vi "Read DMA and Update Waveform.vi"(4 "Delacing Scheme":T3, 6 "Number of Channels":u8, 7 "Timeout?":bool, 8 "error in (no error)":errorcluster, 9 "Total Samples":u32, 10 "Refs in":T1={"Data Type"=enum."Boolean", "DMA_SGL"=refnum, "DMA_U64"=refnum, "DMA_I64"=refnum, "DMA_FXP+/-32.8"=refnum, "DMA_FXP+/-64.32"=refnum, "DMA_U32"=refnum, "DMA_U16"=refnum, "DMA_U8"=refnum, "DMA_I32"=refnum, "DMA_I16"=refnum, "DMA_I8"=refnum, "DMA_FXP+/-32.16"=refnum} {"Data Type" format="%.0x"}, 11 "Multiple Waveforms Write (DBL) in":refnum<class "Multiple Waveforms Write (DBL).lvclass">) -> (0 "error out":errorcluster, 1 "Elements Remaining":u32, 2 "Refs in":T1={"Data Type"=enum."Boolean", "DMA_SGL"=refnum, "DMA_U64"=refnum, "DMA_I64"=refnum, "DMA_FXP+/-32.8"=refnum, "DMA_FXP+/-64.32"=refnum, "DMA_U32"=refnum, "DMA_U16"=refnum, "DMA_U8"=refnum, "DMA_I32"=refnum, "DMA_I16"=refnum, "DMA_I8"=refnum, "DMA_FXP+/-32.16"=refnum} {"Data Type" format="%.0x"}, 3 "Multiple Waveforms Write (DBL) out":refnum<class "Multiple Waveforms Write (DBL).lvclass">)   [LabVIEW 2020, in "FPGA Addon Engine.lvlib"]
uses:
  FPGA Addon Engine.lvlib
  Addon Shared/Types/Delacing Scheme.ctl
  Types/DMA Input Refs.ctl
  Addon Shared/Types/FPGA Addon Data Type.ctl
  <vilib>/NI VeriStand/Custom Device Waveform API/Multiple Waveforms Write (DBL)/Multiple Waveforms Write (DBL).lvclass
  C:/Program Files (x86)/National Instruments/LabVIEW 2020/vi.lib/NI VeriStand/Custom Device Waveform API/Waveform Session.lvclass
  <vilib>/NI VeriStand/Custom Device Waveform API/Waveform Session.lvclass/Waveform Session.ctl
  <vilib>/NI VeriStand/Custom Device Waveform API/Multiple Waveforms Write (DBL)/Multiple Waveforms Write (DBL).lvclass/Multiple Waveforms Write (DBL).ctl
  <vilib>/NI VeriStand/Custom Device Waveform API/Internal Comm Classes/WPL Comm/WPL Comm (2D DBL)/WPL Comm (2D DBL).lvclass/WPL Comm (2D DBL).ctl
  <vilib>/NI VeriStand/Custom Device Waveform API/Internal Comm Classes/WPL Comm/WPL Comm.lvclass/WPL Comm.ctl
  <vilib>/NI VeriStand/Custom Device Waveform API/Multiple Waveforms Write (DBL)/NI VeriStand - Write Multiple Waveforms (DBL).vi
  <vilib>/NI VeriStand/Custom Device Waveform API/Read Sample offset DVR.vi
  <vilib>/NI VeriStand/Custom Device Waveform API/Internal Comm Classes/WPL Comm/WPL Comm (2D DBL)/Comm_write 2d dbl.vi
  <vilib>/NI VeriStand/Custom Device Waveform API/Check Write Size.vi
  <vilib>/NI VeriStand/Custom Device Waveform API/Check Opened.vi
  <vilib>/NI VeriStand/Custom Device Waveform API/Internal Comm Classes/WPL Comm/Direct Send WPL Command.vi
  <vilib>/NI VeriStand/Custom Device Waveform API/Internal Comm Classes/WPL Comm/Convert Q Error to Shutdown Error.vi
  <vilib>/NI VeriStand/Custom Device Waveform API/Internal Comm Classes/WPL Comm/WPL Comm (2D DBL)/WPL Comm (2D DBL).lvclass
  C:/Program Files (x86)/National Instruments/LabVIEW 2020/vi.lib/NI VeriStand/Custom Device Waveform API/Internal Comm Classes/WPL Comm/WPL Comm.lvclass
  <vilib>/Utility/error.llb/Error Cluster From Error Code.vi
  <vilib>/rvi/errors/niLvFpgaAdjustHostInterfaceError.vi
  <vilib>/rvi/interface/nirviMethod/nirviMethod.xnode
  <vilib>/NI VeriStand/Custom Device Waveform API/NI_VS Custom Device Waveform API.lvlib
  <vilib>/FPGAPlugInAG/Dynamic/niLvFpga_ReadFifo_Dynamic.vi
  <vilib>/rvi/errors/niLvFpgaMergeErrorWithErrorCode.vi
  Addon Shared/FPGA Addon Shared.lvlib
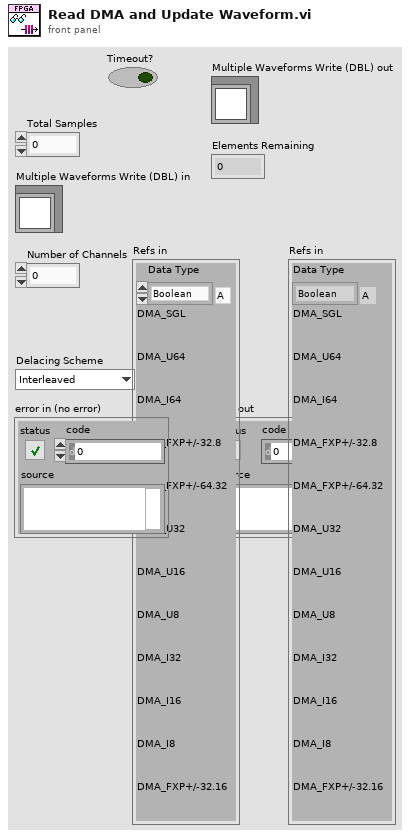
[diagram p1: front panel]
types:
  T1 = typedef "FPGA Addon Engine.lvlib/DMA Input Refs.ctl" = cluster{"Data Type":T2, "DMA_SGL":refnum<k20>, "DMA_U64":refnum<k20>, "DMA_I64":refnum<k20>, "DMA_FXP+/-32.8":refnum<k20>, "DMA_FXP+/-64.32":refnum<k20>, "DMA_U32":refnum<k20>, "DMA_U16":refnum<k20>, "DMA_U8":refnum<k20>, "DMA_I32":refnum<k20>, "DMA_I16":refnum<k20>, "DMA_I8":refnum<k20>, "DMA_FXP+/-32.16":refnum<k20>}
  T2 = typedef "FPGA Addon Shared.lvlib/FPGA Addon Data Type.ctl" = enum8{"<Null>", "I8", "I16", "I32", "I64", "U8", "U16", "U32", "U64", "SGL", "Boolean", "Analog PWM In Settings", "Analog PWM In", "Digital PWM In Settings", "Digital PWM In", "Digital PWM Out", "Sine Out", "FXP", "FXP+/-24.5", "FXP+/-16.5", "FXP+/-32.8", "FXP+/-64.32", "FXP+/-16.7", "FXP+/-20.5", "FXP+/-27.5", "FXP+/-32.16", "FXP+16.3", "FXP+18.3", "Digital Static In", "Digital Static Out", "Digital Static In Settings", "Digital WSS Out", "Quad Encoder Settings", "Quad Encoder In", "Group"}
  T3 = typedef "FPGA Addon Shared.lvlib/Delacing Scheme.ctl" = enum8{"Interleaved", "Bitpacked"}
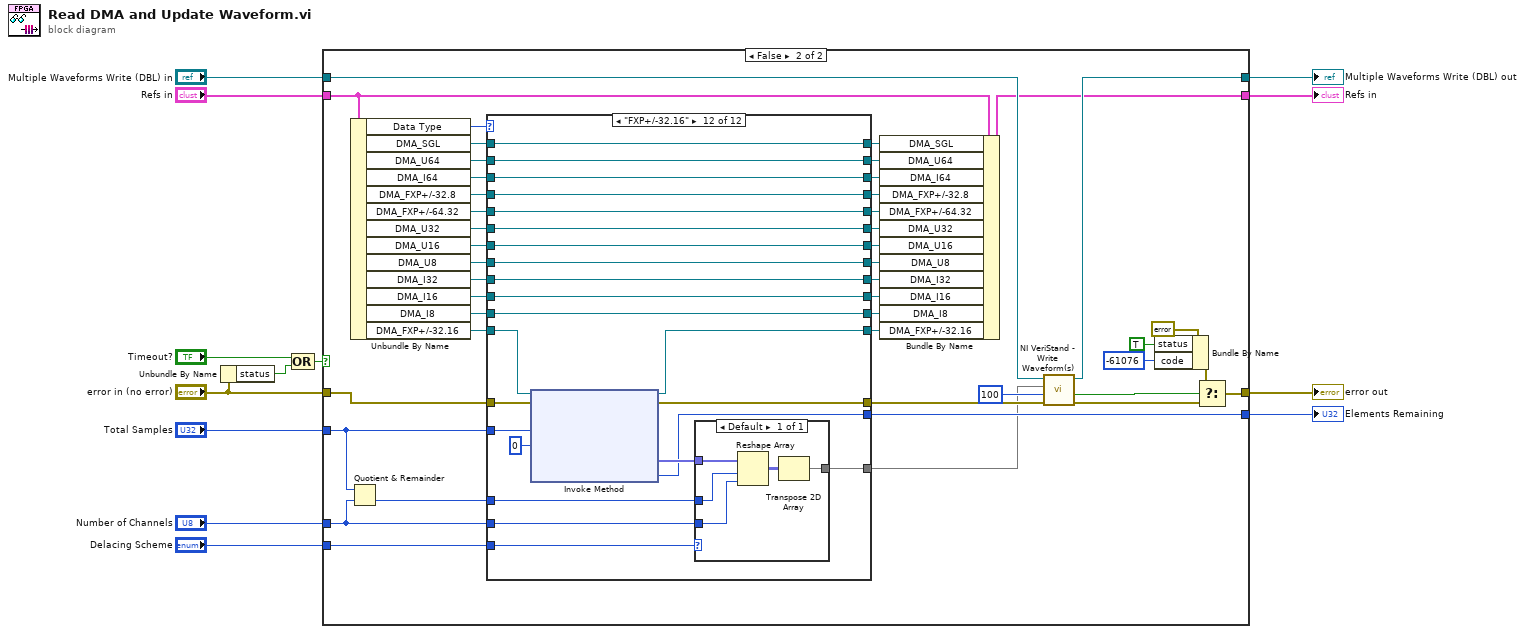
[diagram p0: block diagram]
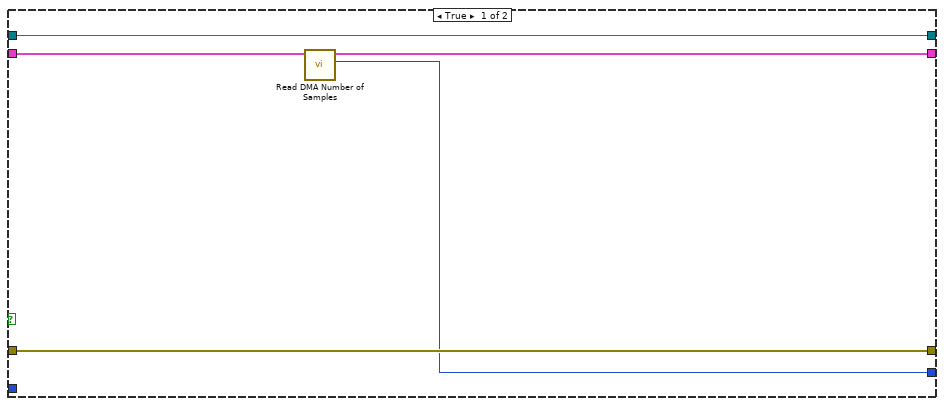
[diagram p2: hidden frame]
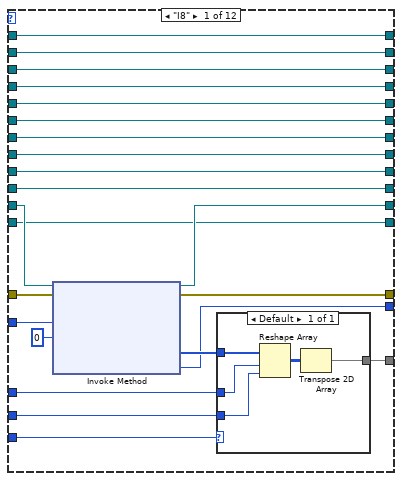
[diagram p3: hidden frame]
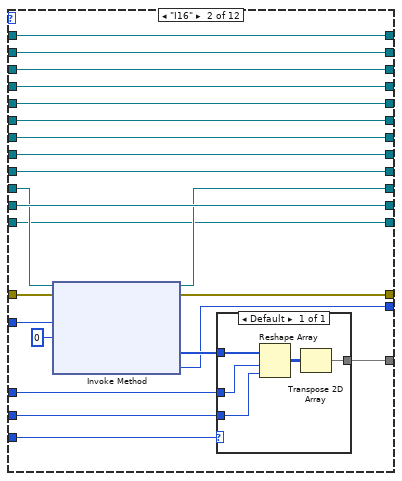
[diagram p4: hidden frame]
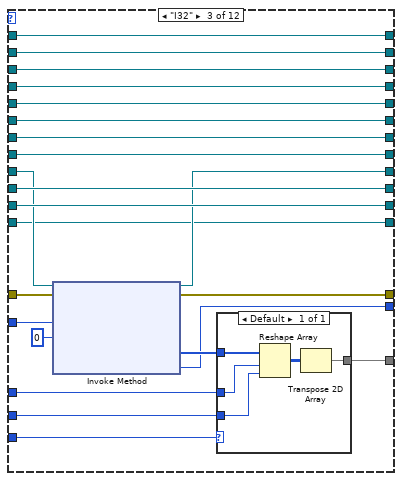
[diagram p5: hidden frame]
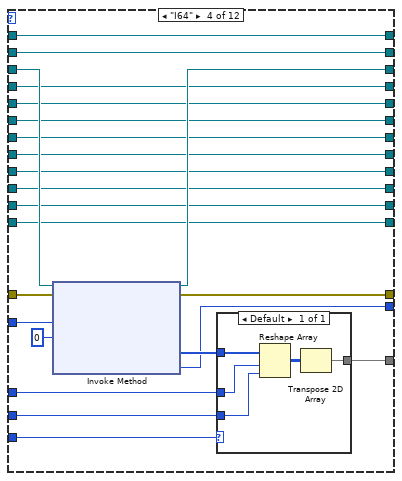
[diagram p6: hidden frame]
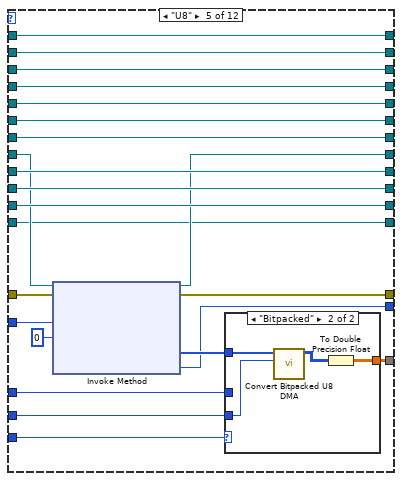
[diagram p7: hidden frame]
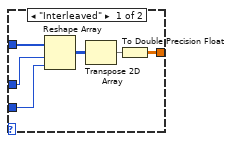
[diagram p8: hidden frame]
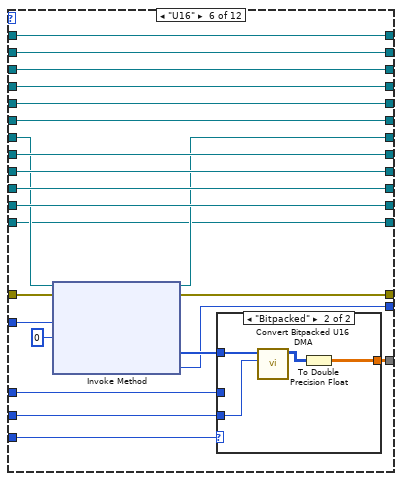
[diagram p9: hidden frame]
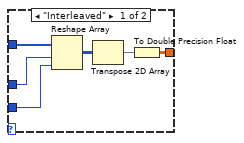
[diagram p10: hidden frame]
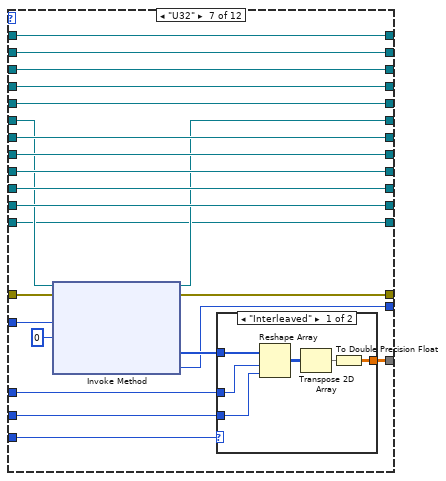
[diagram p11: hidden frame]
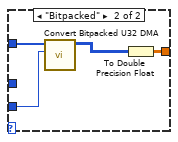
[diagram p12: hidden frame]
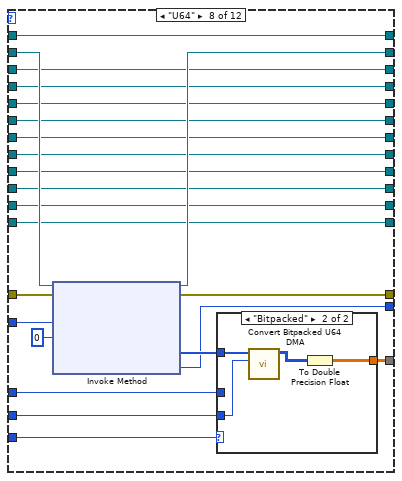
[diagram p13: hidden frame]
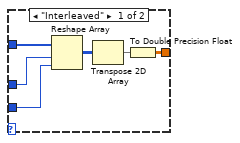
[diagram p14: hidden frame]
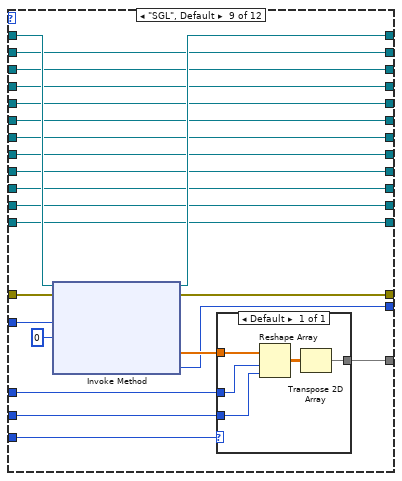
[diagram p15: hidden frame]
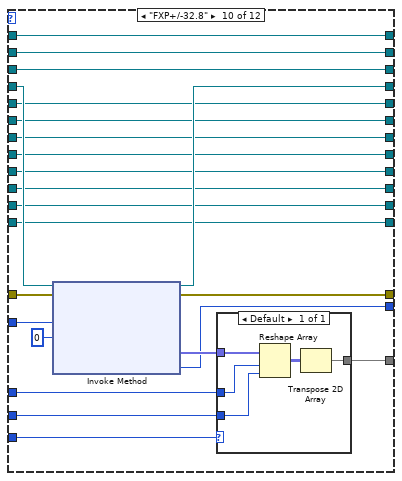
[diagram p16: hidden frame]
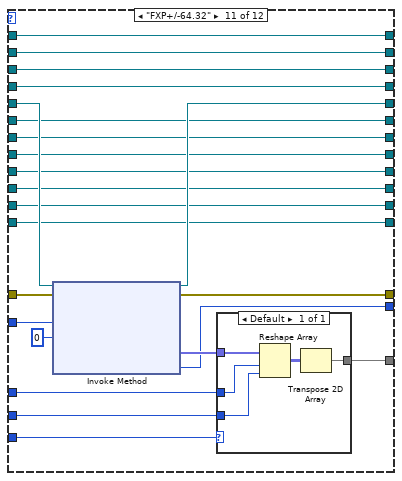
[diagram p17: hidden frame]
diagram:
  n1 = Unbundle By Name("error in (no error)") -> ("status"=w3:bool)
  n2 = Compound Arithmetic op=OR("Timeout?", w3) -> (w1:bool)
  n3 = case shown="False" w1 {
    tunnel: [w17 w63] -> w13
    tunnel: [w16 w56] -> w12
    tunnel: "Delacing Scheme" -> [_ w54]
    tunnel: [w14 w41] -> w10
    tunnel: "Refs in" -> [w15 w42]
    tunnel: [w18 w53] -> w8
    tunnel: "Multiple Waveforms Write (DBL) in" -> [w18 w50]
    tunnel: "Total Samples" -> [_ w49]
    tunnel: "Number of Channels" -> [_ w48]
    tunnel: "error in (no error)" -> [w17 w46]
    frame True {
      n4 = call "Read DMA Number of Samples.vi"("Refs in"=w15) -> ("Elements Remaining"=w16:u32, "Refs out"=w14:T1)  [unwired: 8 in, 1 out]
    }
    frame False {
      n5 = Quotient & Remainder(x=w49, y=w48) -> (floor(x/y)=w47:u32)  [unwired: 1 out]
      n6 = Unbundle By Name(w42) -> ("Data Type"=w45:T2, "DMA_SGL"=w44:refnum<k20>, "DMA_U64"=w43:refnum<k20>, "DMA_I64"=w38:refnum<k20>, "DMA_FXP+/-32.8"=w36:refnum<k20>, "DMA_FXP+/-64.32"=w33:refnum<k20>, "DMA_U32"=w21:refnum<k20>, "DMA_U16"=w24:refnum<k20>, "DMA_U8"=w25:refnum<k20>, "DMA_I32"=w28:refnum<k20>, "DMA_I16"=w29:refnum<k20>, "DMA_I8"=w32:refnum<k20>, "DMA_FXP+/-32.16"=w20:refnum<k20>)
      n7 = case shown="\"FXP+/-32.16\"" w45 {
        tunnel: [w85 w113 w141 w169 w197 w230 w263 w296 w329 w357 w385 w413] -> w56
        tunnel: w54 -> [w84 w112 w140 w168 w196 w229 w262 w295 w328 w356 w384 w412]
        tunnel: [w76 w104 w132 w160 w189 w221 w254 w287 w327 w348 w376 w404] -> w40
        tunnel: [w83 w111 w139 w167 w177 w228 w261 w294 w326 w355 w383 w411] -> w52
        tunnel: [w82 w110 w138 w166 w195 w227 w260 w293 w325 w354 w382 w410] -> w51
        tunnel: w49 -> [w80 w108 w136 w164 w193 w225 w258 w291 w323 w352 w380 w408]
        tunnel: w48 -> [w79 w107 w135 w163 w192 w224 w257 w290 w322 w351 w379 w407]
        tunnel: w47 -> [w78 w106 w134 w162 w191 w223 w256 w289 w321 w350 w378 w406]
        tunnel: w46 -> [w77 w105 w133 w161 w190 w222 w255 w288 w320 w349 w377 w405]
        tunnel: w44 -> [w76 w104 w132 w160 w189 w221 w254 w287 w319 w348 w376 w404]
        tunnel: w43 -> [w67 w95 w123 w157 w180 w212 w245 w286 w318 w347 w375 w403]
        tunnel: [w67 w95 w123 w157 w180 w212 w245 w285 w318 w347 w375 w403] -> w39
        tunnel: w38 -> [w75 w103 w131 w159 w188 w220 w253 w284 w317 w346 w372 w401]
        tunnel: [w75 w103 w131 w158 w188 w220 w253 w284 w317 w346 w372 w401] -> w37
        tunnel: w36 -> [w74 w102 w130 w156 w187 w219 w252 w283 w316 w345 w374 w402]
        tunnel: [w74 w102 w130 w156 w187 w219 w252 w283 w316 w344 w374 w402] -> w35
        tunnel: [w73 w101 w129 w155 w186 w218 w251 w282 w315 w343 w371 w392] -> w34
        tunnel: w33 -> [w73 w101 w129 w155 w186 w218 w251 w282 w315 w343 w373 w392]
        tunnel: w32 -> [w66 w96 w124 w149 w181 w213 w246 w276 w314 w337 w365 w395]
        tunnel: [w65 w96 w124 w149 w181 w213 w246 w276 w314 w337 w365 w395] -> w31
        tunnel: [w68 w93 w125 w150 w182 w214 w247 w277 w313 w338 w366 w396] -> w30
        tunnel: w29 -> [w68 w94 w125 w150 w182 w214 w247 w277 w313 w338 w366 w396]
        tunnel: w28 -> [w69 w97 w122 w151 w183 w215 w248 w278 w312 w339 w367 w397]
        tunnel: [w69 w97 w121 w151 w183 w215 w248 w278 w312 w339 w367 w397] -> w27
        tunnel: [w70 w98 w126 w152 w178 w216 w249 w279 w311 w340 w368 w398] -> w26
        tunnel: w25 -> [w70 w98 w126 w152 w179 w216 w249 w279 w311 w340 w368 w398]
        tunnel: w24 -> [w71 w99 w127 w153 w184 w211 w250 w280 w310 w341 w369 w399]
        tunnel: [w71 w99 w127 w153 w184 w210 w250 w280 w310 w341 w369 w399] -> w23
        tunnel: [w72 w100 w128 w154 w185 w217 w243 w281 w309 w342 w370 w400] -> w22
        tunnel: w21 -> [w72 w100 w128 w154 w185 w217 w244 w281 w309 w342 w370 w400]
        tunnel: w20 -> [w64 w92 w120 w148 w176 w209 w242 w275 w308 w336 w364 w394]
        tunnel: [w64 w92 w120 w148 w176 w209 w242 w275 w308 w336 w364 w393] -> w19
        frame "I8" {
          n8 = xnode "Invoke Method"("FPGA VI Reference In"=w66, "error in"=w77, "Number of Elements"=w80, "Timeout (ms)"=0) -> ("FPGA VI Reference Out"=w65:refnum<k20>, "error out"=w83:errorcluster, "Data"=w86:i8[], "Elements Remaining"=w85:u32)
          n9 = case shown="Default" w84 {
            tunnel: w86 -> [w90]
            tunnel: [w89] -> w82
            tunnel: w79 -> [w88]
            tunnel: w78 -> [w87]
            frame Default {
              n10 = Reshape Array(w90, w87, w88) -> (w91:i8[][])
              n11 = Transpose 2D Array(2D array=w91) -> (transposed array=w89:i8[][])
            }
          }
        }
        frame "I16" {
          n12 = xnode "Invoke Method"("FPGA VI Reference In"=w94, "error in"=w105, "Number of Elements"=w108, "Timeout (ms)"=0) -> ("FPGA VI Reference Out"=w93:refnum<k20>, "error out"=w111:errorcluster, "Data"=w114:i16[], "Elements Remaining"=w113:u32)
          n13 = case shown="Default" w112 {
            tunnel: w114 -> [w118]
            tunnel: [w117] -> w110
            tunnel: w107 -> [w116]
            tunnel: w106 -> [w115]
            frame Default {
              n14 = Reshape Array(w118, w115, w116) -> (w119:i16[][])
              n15 = Transpose 2D Array(2D array=w119) -> (transposed array=w117:i16[][])
            }
          }
        }
        frame "I32" {
          n16 = xnode "Invoke Method"("FPGA VI Reference In"=w122, "error in"=w133, "Number of Elements"=w136, "Timeout (ms)"=0) -> ("FPGA VI Reference Out"=w121:refnum<k20>, "error out"=w139:errorcluster, "Data"=w142:i32[], "Elements Remaining"=w141:u32)
          n17 = case shown="Default" w140 {
            tunnel: w142 -> [w146]
            tunnel: [w145] -> w138
            tunnel: w135 -> [w144]
            tunnel: w134 -> [w143]
            frame Default {
              n18 = Reshape Array(w146, w143, w144) -> (w147:i32[][])
              n19 = Transpose 2D Array(2D array=w147) -> (transposed array=w145:i32[][])
            }
          }
        }
        frame "I64" {
          n20 = xnode "Invoke Method"("FPGA VI Reference In"=w159, "error in"=w161, "Number of Elements"=w164, "Timeout (ms)"=0) -> ("FPGA VI Reference Out"=w158:refnum<k20>, "error out"=w167:errorcluster, "Data"=w170:i64[], "Elements Remaining"=w169:u32)
          n21 = case shown="Default" w168 {
            tunnel: w170 -> [w174]
            tunnel: [w173] -> w166
            tunnel: w163 -> [w172]
            tunnel: w162 -> [w171]
            frame Default {
              n22 = Reshape Array(w174, w171, w172) -> (w175:i64[][])
              n23 = Transpose 2D Array(2D array=w175) -> (transposed array=w173:i64[][])
            }
          }
        }
        frame "U8" {
          n24 = xnode "Invoke Method"("FPGA VI Reference In"=w179, "error in"=w190, "Number of Elements"=w193, "Timeout (ms)"=0) -> ("FPGA VI Reference Out"=w178:refnum<k20>, "error out"=w177:errorcluster, "Data"=w198:u8[], "Elements Remaining"=w197:u32)
          n25 = case shown="\"Bitpacked\"" w196 {
            tunnel: w198 -> [w203 w208]
            tunnel: [w199 w205] -> w195
            tunnel: w192 -> [w201 w206]
            tunnel: w191 -> [w200 _]
            frame "Interleaved" {
              n26 = Reshape Array(w203, w200, w201) -> (w204:u8[][])
              n27 = Transpose 2D Array(2D array=w204) -> (transposed array=w202:u8[][])
              n28 = To Double Precision Float(number=w202) -> (double precision float=w199:dbl[][])
            }
            frame "Bitpacked" {
              n29 = call "Convert Bitpacked U8 DMA.vi"("Channels"=w206, "binary array"=w208) -> ("Data"=w207:u8[][])  [unwired: 9 in]
              n30 = To Double Precision Float(number=w207) -> (double precision float=w205:dbl[][])
            }
          }
        }
        frame "U16" {
          n31 = xnode "Invoke Method"("FPGA VI Reference In"=w211, "error in"=w222, "Number of Elements"=w225, "Timeout (ms)"=0) -> ("FPGA VI Reference Out"=w210:refnum<k20>, "error out"=w228:errorcluster, "Data"=w231:u16[], "Elements Remaining"=w230:u32)
          n32 = case shown="\"Bitpacked\"" w229 {
            tunnel: w231 -> [w236 w241]
            tunnel: [w232 w239] -> w227
            tunnel: w224 -> [w234 w238]
            tunnel: w223 -> [w233 _]
            frame "Interleaved" {
              n33 = Reshape Array(w236, w233, w234) -> (w237:u16[][])
              n34 = Transpose 2D Array(2D array=w237) -> (transposed array=w235:u16[][])
              n35 = To Double Precision Float(number=w235) -> (double precision float=w232:dbl[][])
            }
            frame "Bitpacked" {
              n36 = call "Convert Bitpacked U16 DMA.vi"("Channels"=w238, "binary array"=w241) -> ("Data"=w240:u8[][])  [unwired: 9 in]
              n37 = To Double Precision Float(number=w240) -> (double precision float=w239:dbl[][])
            }
          }
        }
        frame "U32" {
          n38 = xnode "Invoke Method"("FPGA VI Reference In"=w244, "error in"=w255, "Number of Elements"=w258, "Timeout (ms)"=0) -> ("FPGA VI Reference Out"=w243:refnum<k20>, "error out"=w261:errorcluster, "Data"=w264:u32[], "Elements Remaining"=w263:u32)
          n39 = case shown="\"Interleaved\"" w262 {
            tunnel: w264 -> [w269 w273]
            tunnel: [w265 w274] -> w260
            tunnel: w257 -> [w267 w272]
            tunnel: w256 -> [w266 _]
            frame "Interleaved" {
              n40 = Reshape Array(w269, w266, w267) -> (w270:u32[][])
              n41 = Transpose 2D Array(2D array=w270) -> (transposed array=w268:u32[][])
              n42 = To Double Precision Float(number=w268) -> (double precision float=w265:dbl[][])
            }
            frame "Bitpacked" {
              n43 = call "Convert Bitpacked U32 DMA.vi"("Channels"=w272, "binary array"=w273) -> ("Data"=w271:u8[][])  [unwired: 9 in]
              n44 = To Double Precision Float(number=w271) -> (double precision float=w274:dbl[][])
            }
          }
        }
        frame "U64" {
          n45 = xnode "Invoke Method"("FPGA VI Reference In"=w286, "error in"=w288, "Number of Elements"=w291, "Timeout (ms)"=0) -> ("FPGA VI Reference Out"=w285:refnum<k20>, "error out"=w294:errorcluster, "Data"=w297:u64[], "Elements Remaining"=w296:u32)
          n46 = case shown="\"Bitpacked\"" w295 {
            tunnel: w297 -> [w302 w307]
            tunnel: [w298 w304] -> w293
            tunnel: w290 -> [w301 w306]
            tunnel: w289 -> [w300 _]
            frame "Interleaved" {
              n47 = Reshape Array(w302, w300, w301) -> (w303:u64[][])
              n48 = Transpose 2D Array(2D array=w303) -> (transposed array=w299:u64[][])
              n49 = To Double Precision Float(number=w299) -> (double precision float=w298:dbl[][])
            }
            frame "Bitpacked" {
              n50 = call "Convert Bitpacked U64 DMA.vi"("Channels"=w306, "binary array"=w307) -> ("Data"=w305:u8[][])  [unwired: 9 in]
              n51 = To Double Precision Float(number=w305) -> (double precision float=w304:dbl[][])
            }
          }
        }
        frame "SGL", Default {
          n52 = xnode "Invoke Method"("FPGA VI Reference In"=w319, "error in"=w320, "Number of Elements"=w323, "Timeout (ms)"=0) -> ("FPGA VI Reference Out"=w327:refnum<k20>, "error out"=w326:errorcluster, "Data"=w330:sgl[], "Elements Remaining"=w329:u32)
          n53 = case shown="Default" w328 {
            tunnel: w330 -> [w334]
            tunnel: [w333] -> w325
            tunnel: w322 -> [w332]
            tunnel: w321 -> [w331]
            frame Default {
              n54 = Reshape Array(w334, w331, w332) -> (w335:sgl[][])
              n55 = Transpose 2D Array(2D array=w335) -> (transposed array=w333:sgl[][])
            }
          }
        }
        frame "FXP+/-32.8" {
          n56 = xnode "Invoke Method"("FPGA VI Reference In"=w345, "error in"=w349, "Number of Elements"=w352, "Timeout (ms)"=0) -> ("FPGA VI Reference Out"=w344:refnum<k20>, "error out"=w355:errorcluster, "Data"=w358:fxp<+/-,32,8>[], "Elements Remaining"=w357:u32)
          n57 = case shown="Default" w356 {
            tunnel: w358 -> [w362]
            tunnel: [w361] -> w354
            tunnel: w351 -> [w360]
            tunnel: w350 -> [w359]
            frame Default {
              n58 = Reshape Array(w362, w359, w360) -> (w363:fxp<+/-,32,8>[][])
              n59 = Transpose 2D Array(2D array=w363) -> (transposed array=w361:fxp<+/-,32,8>[][])
            }
          }
        }
        frame "FXP+/-64.32" {
          n60 = xnode "Invoke Method"("FPGA VI Reference In"=w373, "error in"=w377, "Number of Elements"=w380, "Timeout (ms)"=0) -> ("FPGA VI Reference Out"=w371:refnum<k20>, "error out"=w383:errorcluster, "Data"=w386:fxp<+/-,64,32>[], "Elements Remaining"=w385:u32)
          n61 = case shown="Default" w384 {
            tunnel: w386 -> [w390]
            tunnel: [w389] -> w382
            tunnel: w379 -> [w388]
            tunnel: w378 -> [w387]
            frame Default {
              n62 = Reshape Array(w390, w387, w388) -> (w391:fxp<+/-,64,32>[][])
              n63 = Transpose 2D Array(2D array=w391) -> (transposed array=w389:fxp<+/-,64,32>[][])
            }
          }
        }
        frame "FXP+/-32.16" {
          n64 = xnode "Invoke Method"("FPGA VI Reference In"=w394, "error in"=w405, "Number of Elements"=w408, "Timeout (ms)"=0) -> ("FPGA VI Reference Out"=w393:refnum<k20>, "error out"=w411:errorcluster, "Data"=w414:fxp<+/-,32,16>[], "Elements Remaining"=w413:u32)
          n65 = case shown="Default" w412 {
            tunnel: w414 -> [w418]
            tunnel: [w417] -> w410
            tunnel: w407 -> [w416]
            tunnel: w406 -> [w415]
            frame Default {
              n66 = Reshape Array(w418, w415, w416) -> (w419:fxp<+/-,32,16>[][])
              n67 = Transpose 2D Array(2D array=w419) -> (transposed array=w417:fxp<+/-,32,16>[][])
            }
          }
        }
      }
      n68 = Bundle By Name(cluster=w42, "DMA_SGL"=w40, "DMA_U64"=w39, "DMA_I64"=w37, "DMA_FXP+/-32.8"=w35, "DMA_FXP+/-64.32"=w34, "DMA_U32"=w22, "DMA_U16"=w23, "DMA_U8"=w26, "DMA_I32"=w27, "DMA_I16"=w30, "DMA_I8"=w31, "DMA_FXP+/-32.16"=w19) -> (w41:T1)
      n69 = call-poly <vilib>:"NI VeriStand - Write Waveform(s).vi"("error in (no error)"=w52, "timeout in ms (0)"=100, "Data"=w51, "Multiple Waveforms Write Session (DBL) in"=w50) -> ("error out"=w62:errorcluster, "timed out?"=w57:bool, "Multiple Waveforms Write Session (DBL) out"=w53:refnum<class "Multiple Waveforms Write (DBL).lvclass">)  [unwired: 5 in]
      n70 = Bundle By Name(cluster=errorcluster {"status"=FALSE, "code"=0, "source"=""} ("input cluster"), "status"=TRUE, "code"=-61076) -> (w61:errorcluster)
      n71 = Select(t=w61, s=w57, f=w62) -> (s? t:f=w63:errorcluster)
    }
  }
  "error out" <- w13
  "Elements Remaining" <- w12
  "Refs in" <- w10
  "Multiple Waveforms Write (DBL) out" <- w8
